vi "SetCurRecordColorTo2DListCtrl.vi"(9 "color":u32(colorbox)=16711680, 10 "column index":u16, 11 "multiple list in":refnum<vi>) -> (3 "multiple list out":refnum<vi>)   [LabVIEW 2018, in "Library-Ctrl.lvlib"]
uses:
  Library-Ctrl.lvlib
  <vilib>/Utility/miscctls.llb/LVRowAndColumnTypeDef.ctl
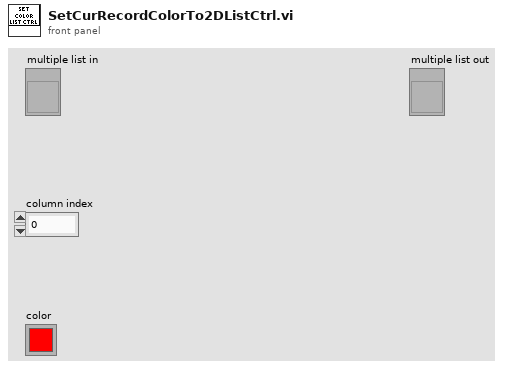
[diagram p1: front panel]
types:
  T1 = typedef "LVRowAndColumnTypeDef.ctl" = cluster{"Row":i32, "Column":i32}
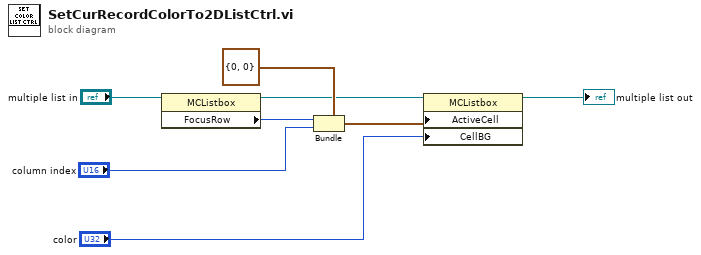
[diagram p0: block diagram]
diagram:
  n1 = property class="MCListbox"(reference="multiple list in") -> (reference out=w4:refnum<vi>, "FocusRow"=w6:i32)  [unwired: 1 in, 1 out]
  n2 = Bundle(cluster=T1 {"Row"=0, "Column"=0} ("활성 셀:활성 셀"), "Row"=w6, "Column"="column index") -> (w3:T1)
  n3 = property class="MCListbox"(reference=w4, "ActiveCell"=w3, "CellBG"="color") -> (reference out=→"multiple list out":refnum<vi>)  [unwired: 1 in, 1 out]
